vi "EditorThumbnail continueShiftArray.vi"(8 "error in (no error)":errorcluster, 11 "EditorThumbnail in":refnum<class "EditorThumbnail.lvclass">) -> (0 "error out":errorcluster, 2 "Timing":bool, 3 "EditorThumbnail out":refnum<class "EditorThumbnail.lvclass">)   [LabVIEW 2018, in "EditorThumbnail.lvclass"]
uses:
  EditorThumbnail.lvclass
  EditorThumbnail.lvclass/EditorThumbnail.ctl
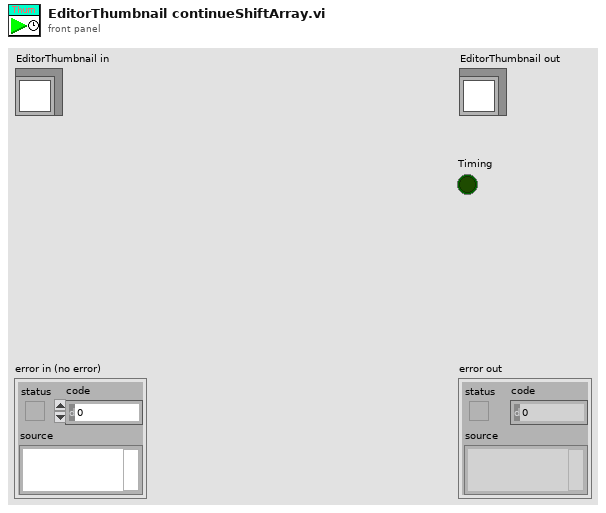
[diagram p1: front panel]
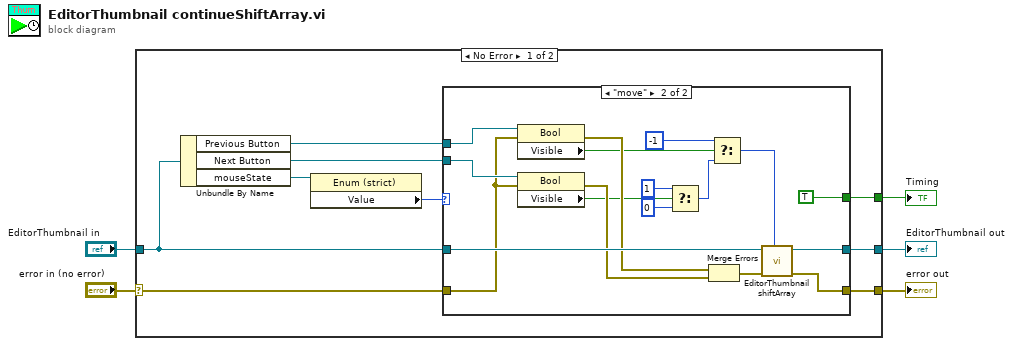
[diagram p0: block diagram]
diagram:
  n1 = case shown="No Error" "error in (no error)" {
    selector: "error in (no error)" -> [w8 w35]
    tunnel: [w7 w35] -> w4
    tunnel: [w6 w34] -> w2
    tunnel: "EditorThumbnail in" -> [w9 w34]
    tunnel: [w12 _] -> w1
    frame No Error {
      n2 = Unbundle By Name(w9) -> ("Previous Button"=w11:refnum<vi>, "Next Button"=w10:refnum<vi>, "mouseState"=w14:refnum<vi>)
      n3 = property class="Enum (strict)"(reference=w14) -> ("Value"=w13:enum16{"idle", "down", "move", "up"})  [unwired: 1 in, 2 out]
      n4 = case shown="\"move\"" w13 {
        tunnel: [_ TRUE] -> w12
        tunnel: w11 -> [_ w32]
        tunnel: w10 -> [_ w31]
        tunnel: w9 -> [w15 w30]
        tunnel: w8 -> [w16 w29]
        tunnel: [w16 w25] -> w7
        tunnel: [w15 w17] -> w6
        frame "idle", Default {
        }
        frame "move" {
          n5 = property class="Bool"(reference=w32, error in=w29) -> (error out=w28:errorcluster, "Visible"=w24:bool)  [unwired: 1 out]
          n6 = property class="Bool"(reference=w31, error in=w29) -> (error out=w27:errorcluster, "Visible"=w22:bool)  [unwired: 1 out]
          n7 = Select(t=1 ("add"), s=w22, f=0) -> (s? t:f=w19:i32)
          n8 = Merge Errors(w28, w27) -> (w26:errorcluster)
          n9 = Select(t=-1 ("add"), s=w24, f=w19) -> (s? t:f=w18:i32)
          n10 = call "EditorThumbnail shiftArray.vi"("add"=w18, "error in (no error)"=w26, "EditorThumbnail in"=w30) -> ("error out"=w25:errorcluster, "EditorThumbnail out"=w17:refnum<class "EditorThumbnail.lvclass">)  [unwired: 7 in]
        }
      }
    }
    frame Error {
    }
  }
  "error out" <- w4
  "EditorThumbnail out" <- w2
  "Timing" <- w1
